vi "Fit Multi-Gaus Peaks.vi"(4 "Use last fit as  guess":bool, 5 "Window end":dbl=697.0, 6 "Repeat":i32, 7 "Window start":dbl=690.0, 8 "Error In":errorcluster, 9 "Fit parameters":T1={"Peaks"=[{"Amplitude"=4000.0, "Center"=694.3, "Width"=0.4}, {"Amplitude"=2000.0, "Center"=692.8, "Width"=0.4}], "Slope"=0.0, "Intercept"=0.0, "Function"=enum."Gauss"}, 10 "Y":dbl[](array[numeric]), 11 "X":dbl[](array[numeric])) -> (0 "Error Out":errorcluster, 1 "Fit parameters out":T1={"Peaks"=[{"Amplitude"=4000.0, "Center"=694.3, "Width"=0.4}, {"Amplitude"=2000.0, "Center"=692.8, "Width"=0.4}], "Slope"=nan, "Intercept"=0.0, "Function"=enum."Gauss"}, 2 "Fit plot":cluster{"Array":dbl[], "Array":dbl[]})   [LabVIEW 2016]
uses:
  Multi-peak Parameters.ctl
  Peak Parameters.ctl
  Smooth Background DBL.vi
  <vilib>/Analysis/NI_AALPro.lvlib
panel:
  out "errors":i32[](array[numeric])
  in  "Filter background":bool
  out "XY Graph":cluster{"all rows":dbl[], "Data out":dbl[]}[](graph)
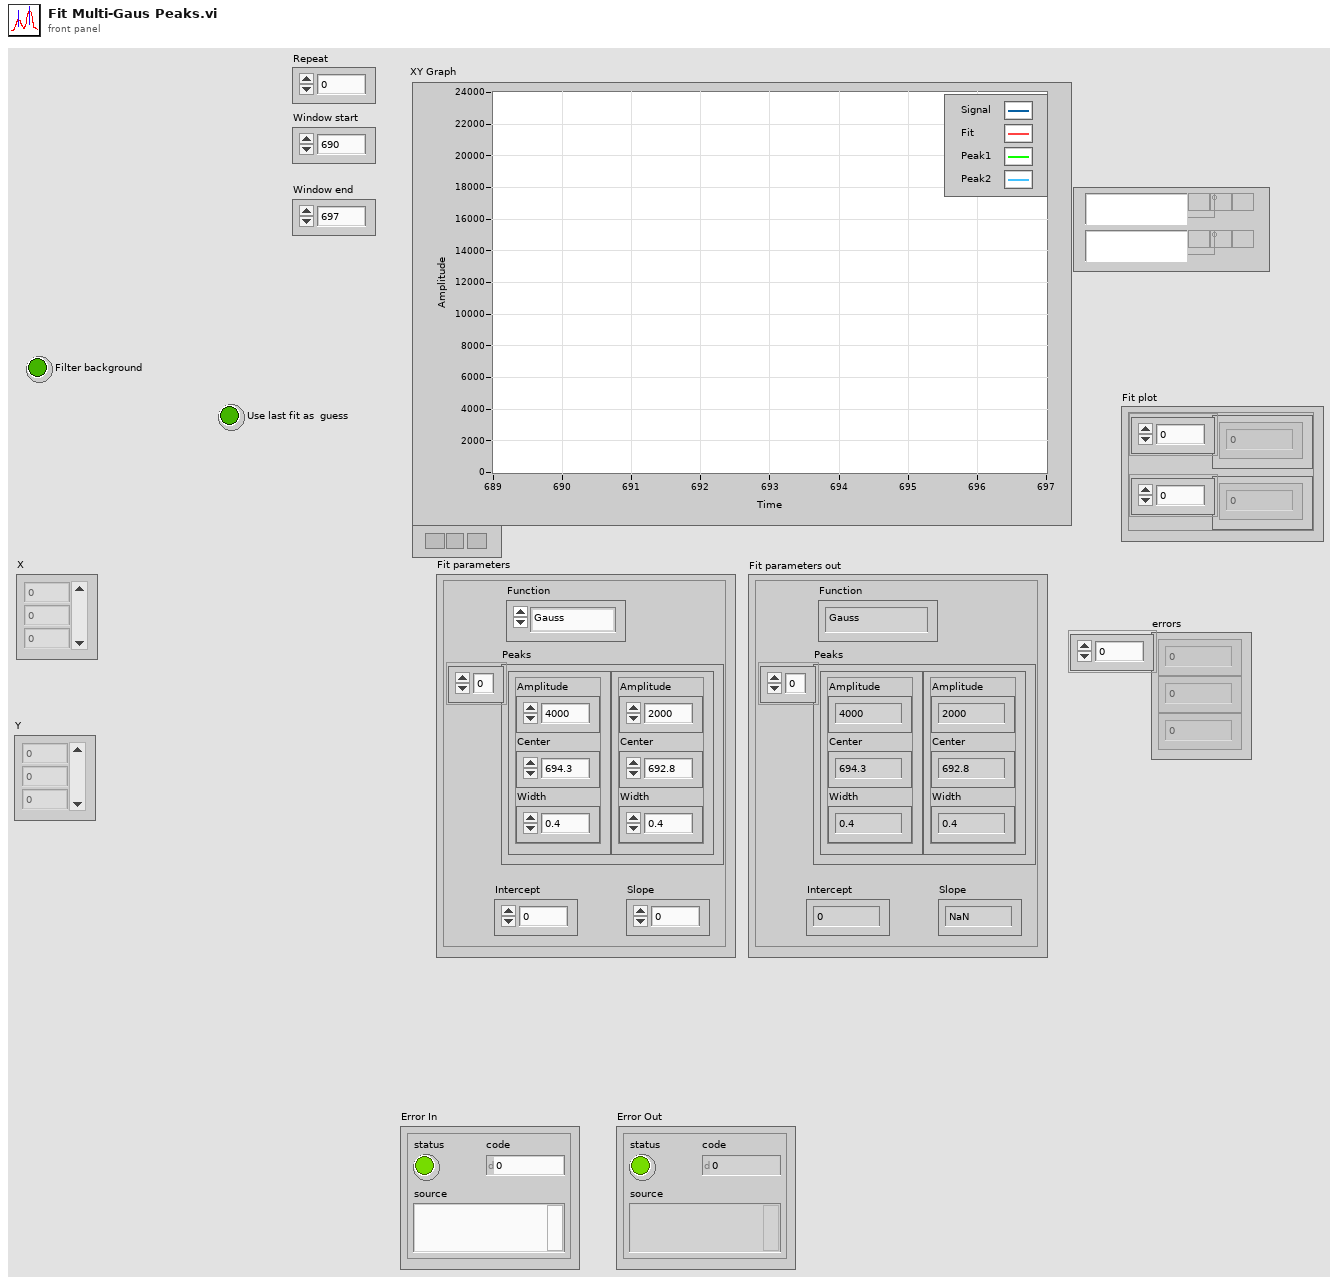
[diagram p1: front panel]
types:
  T1 = typedef "Multi-peak Parameters.ctl" = cluster{"Peaks":T2[], "Slope":dbl, "Intercept":dbl, "Function":enum16{"Gauss", "Lorentz"}}
  T2 = typedef "Peak Parameters.ctl" = cluster{"Amplitude":dbl, "Center":dbl, "Width":dbl}
  T3 = cluster{"amp min":dbl, "amp max":dbl, "center min":dbl, "center max":dbl, "deviation min":dbl, "deviation max":dbl, "offset min":dbl, "offset max":dbl}
  T4 = enum16{"Lowpass", "Highpass", "Bandpass", "Bandstop"}
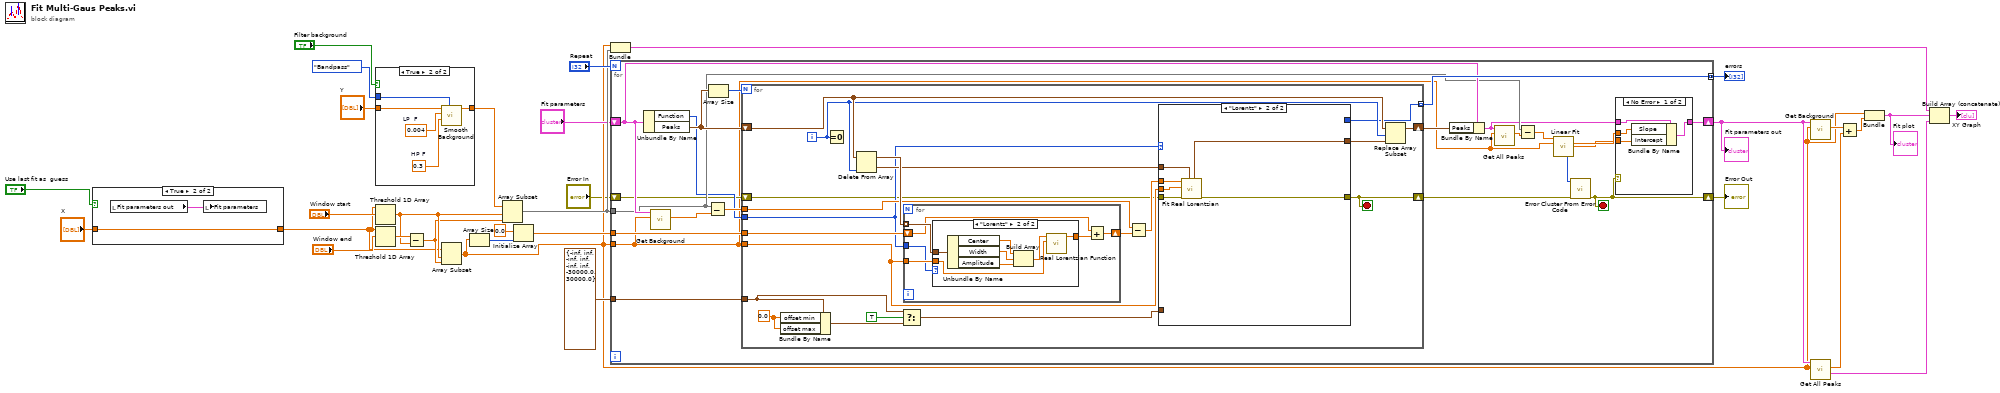
[diagram p0: block diagram]
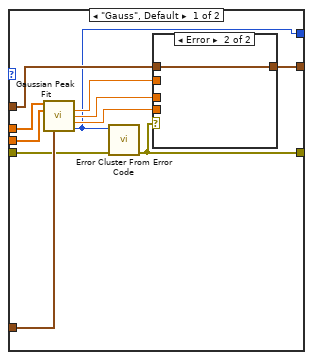
[diagram p4: hidden frame]
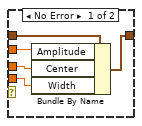
[diagram p5: hidden frame]
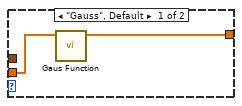
[diagram p6: hidden frame]
diagram:
  n1 = case shown="True" "Use last fit as  guess" {
    tunnel: "X" -> [w32 w34]
    tunnel: [w32 w34] -> w10
    frame False {
    }
    frame True {
      n2 = local read "Fit parameters out"() -> (w33:T1)
      n3 = local write "Fit parameters"(w33) -> ()
    }
  }
  n4 = case shown="True" "Filter background" {
    tunnel: T4."Bandpass" ("Type") -> [_ w40]
    tunnel: "Y" -> [w35 w37]
    tunnel: [w35 w36] -> w25
    frame False {
    }
    frame True {
      w38 = 0.3  # HP F
      w39 = 0.004  # LP  F
      n5 = call-poly "Smooth Background.vi"("Type"=w40, "HP F"=w38, "LP  F"=w39, "Data"=w37) -> ("Data out"=w36:dbl[])  [unwired: 6 in, 1 out]
    }
  }
  n6 = Threshold 1D Array(2:"Window start", 3:w10) -> (0:w27:dbl)  [unwired: 1 in]
  n7 = Threshold 1D Array(2:"Window end", 3:w10) -> (0:w28:dbl)  [unwired: 1 in]
  n8 = Subtract(x=w28, y=w27) -> (x-y=w26:dbl)
  n9 = Array Subset(array=w10, index=w27, length=w26) -> (w3:dbl[])
  n10 = Array Size(array=w3) -> (size(s)=w21:i32)
  n11 = Array Subset(array=w25, index=w27, length=w26) -> (w15:dbl[])
  n12 = Initialize Array(0.0 ("element"), w21) -> (w17:dbl[])
  n13 = Bundle(w3, w15) -> (w29:cluster{dbl[], dbl[]})  [unwired: 1 in]
  n14 = for {
    N: "Repeat" -> [_]
    tunnel: w3 -> [w45]
    tunnel: w17 -> [w61]
    tunnel: w15 -> [w49]
    tunnel: T3 {"amp min"=-inf, "amp max"=inf, "center min"=-inf, "center max"=inf, "deviation min"=-inf, "deviation max"=inf, "offset min"=-30000.0, "offset max"=30000.0} ("parameter bounds") -> [w60]
    tunnel: [w59] -> w14 mode=concatenating
    shift-right: [w56] -> w6
    shift-left: "Fit parameters" -> [w52]
    shift-right: [w42] -> w1
    shift-left: "Error In" -> [w46]
    stop <- w42 stop-if-true
    n15 = Unbundle By Name(w52) -> ("Function"=w47:enum16{"Gauss", "Lorentz"}, "Peaks"=w53:T2[])
    n16 = call "Get Background.vi"("X"=w45, "Fit parameters"=w52) -> ("Y"=w55:dbl[])  [unwired: 9 in]
    n17 = Subtract(x=w49, y=w55) -> (x-y=w54:dbl[])
    n18 = Array Size(array=w53) -> (size(s)=w62:i32)
    n19 = for {
      N: w62 -> [_]
      tunnel: w45 -> [w71]
      tunnel: w61 -> [w86]
      tunnel: w54 -> [w84]
      shift-right: [w79] -> w51
      shift-left: w53 -> [w82]
      tunnel: w60 -> [w77]
      tunnel: [w73] -> w59 mode=indexing
      tunnel: w47 -> [w70]
      shift-right: [w68] -> w43
      shift-left: w46 -> [w69]
      i -> [w78]
      stop <- w68 stop-if-true
      w74 = 0.0
      n20 = Bundle By Name(cluster=w77, "offset min"=w74, "offset max"=w74) -> (w76:T3)
      n21 = Equal To 0?(x=w78) -> ()  [unwired: 1 out]
      n22 = Delete From Array(array=w82, index=w78) -> (deleted portion=w81:T2, array with subset deleted=w87:T2[])  [unwired: 1 in]
      n23 = Select(t=w77, s=TRUE, f=w76) -> (s? t:f=w75:T3)
      n24 = for {
        tunnel: w87 -> [w116] mode=indexing
        tunnel: w71 -> [w115]
        shift-right: [w112] -> w85
        shift-left: w86 -> [w114]
        tunnel: w70 -> [w111]
        n25 = case shown="\"Lorentz\"" w111 {
          tunnel: w116 -> [_ w122]
          tunnel: w115 -> [w118 w119]
          tunnel: [w117 w121] -> w113
          frame "Gauss", Default {
            n26 = call "Gaus Function.vi"("X"=w118) -> ("Y"=w117:dbl[])  [unwired: 10 in]
          }
          frame "Lorentz" {
            n27 = Unbundle By Name(w122) -> ("Center"=w125:dbl, "Width"=w124:dbl, "Amplitude"=w123:dbl)
            n28 = Build Array(w125, w124, w123) -> (w120:dbl[])
            n29 = call "Real Lorentzian Function.vi"("X"=w119, "a"=w120) -> ("f(X,a)"=w121:dbl[])  [unwired: 2 in, 2 out]
          }
        }
        n30 = Add(x=w114, y=w113) -> (x+y=w112:dbl[])
      }
      n31 = Subtract(x=w84, y=w85) -> (x-y=w83:dbl[])
      n32 = case shown="\"Lorentz\"" w70 {
        tunnel: w83 -> [w98 w110]
        tunnel: w81 -> [w91 w107]
        tunnel: [w92 w108] -> w80
        tunnel: w75 -> [w94 _]
        tunnel: [w90 _] -> w73
        tunnel: w71 -> [w93 w109]
        tunnel: w69 -> [w89 w106]
        tunnel: [w88 w105] -> w68
        frame "Gauss", Default {
          n33 = call <vilib>:"Gaussian Peak Fit.vi"("Y"=w98, "X"=w93, "parameter bounds"=w94) -> ("amplitude"=w97:dbl, "center"=w96:dbl, "standard deviation"=w95:dbl, "error"=w90:i32)  [unwired: 6 in, 3 out]
          n34 = call <vilib>:"Error Cluster From Error Code.vi"("error in (no error)"=w89, "error code (0)"=w90) -> ("error out"=w88:errorcluster)  [unwired: 7 in]
          n35 = case shown="Error" w88 {
            tunnel: w97 -> [w103 _]
            tunnel: w96 -> [w102 _]
            tunnel: w95 -> [w101 _]
            tunnel: [w100 w104] -> w92
            tunnel: w91 -> [w99 w104]
            frame No Error {
              n36 = Bundle By Name(cluster=w99, "Amplitude"=w103, "Center"=w102, "Width"=w101) -> (w100:T2)
            }
            frame Error {
            }
          }
        }
        frame "Lorentz" {
          n37 = call "Fit Real Lorentzian.vi"("Initial guess"=w107, "Error In"=w106, "X"=w109, "Y"=w110) -> ("Error Out"=w105:errorcluster, "Fit"=w108:T2)  [unwired: 6 in]
        }
      }
      n38 = Replace Array Subset(array=w82, new element=w80, index=w78) -> (w79:T2[])
    }
    n39 = Bundle By Name(cluster=w52, "Peaks"=w51) -> (w41:T1)
    n40 = call "Get All Peaks.vi"("X"=w45, "Fit parameters"=w41) -> ("Y"=w50:dbl[])  [unwired: 8 in, 1 out]
    n41 = Subtract(x=w49, y=w50) -> (x-y=w48:dbl[])
    n42 = call <vilib>:"Linear Fit.vi"("Y"=w48, "X"=w45) -> ("slope"=w58:dbl, "intercept"=w57:dbl, "error"=w44:i32)  [unwired: 9 in, 2 out]
    n43 = call <vilib>:"Error Cluster From Error Code.vi"("error in (no error)"=w43, "error code (0)"=w44) -> ("error out"=w42:errorcluster)  [unwired: 7 in]
    n44 = case shown="No Error" w42 {
      tunnel: w58 -> [w66 _]
      tunnel: w57 -> [w65 _]
      tunnel: [w64 w67] -> w56
      tunnel: w41 -> [w63 w67]
      frame No Error {
        n45 = Bundle By Name(cluster=w63, "Slope"=w66, "Intercept"=w65) -> (w64:T1)
      }
      frame Error {
      }
    }
  }
  "errors" <- w14
  "Fit parameters out" <- w6
  "Error Out" <- w1
  n46 = call "Get Background.vi"("X"=w3, "Fit parameters"=w6) -> ("Y"=w7:dbl[])  [unwired: 9 in]
  n47 = call "Get All Peaks.vi"("X"=w3, "Fit parameters"=w6) -> ("Individual plots"=w5:cluster{"X":dbl[], "f(X,a)":dbl[]}[], "Y"=w4:dbl[])  [unwired: 8 in]
  n48 = Add(x=w7, y=w4) -> (x+y=w9:dbl[])
  n49 = Bundle(w3, w9) -> (w16:cluster{dbl[], dbl[]})  [unwired: 1 in]
  "Fit plot" <- w16
  n50 = Build Array (concatenate)(w29, w16, w5) -> (→"XY Graph":cluster{"X":dbl[], "f(X,a)":dbl[]}[])
